vi "SHA256_hash.vi"(8 "error in (no error)":errorcluster, 11 "text in":string) -> (0 "error out":errorcluster, 3 "hash out":string)   [LabVIEW 2020]
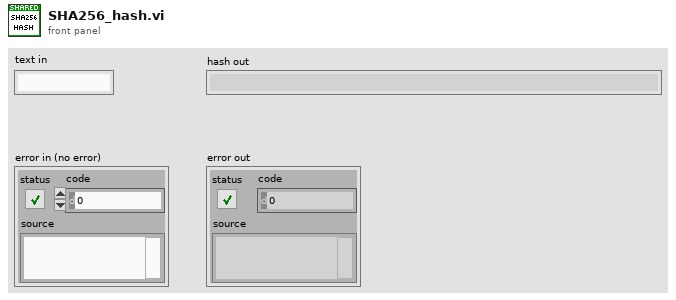
[diagram p1: front panel]
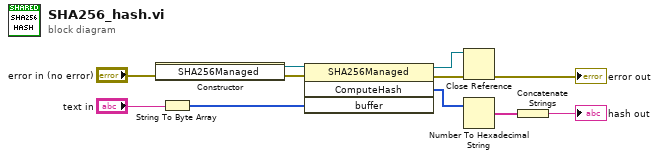
[diagram p0: block diagram]
diagram:
  n1 = constructor class="SHA256Managed"(error in="error in (no error)") -> (reference out=w9:refnum<k24>, error out=w8:errorcluster)  [unwired: 2 in, 1 out]
  n2 = String To Byte Array(string="text in") -> (unsigned byte array=w6:u8[])
  n3 = invoke class="SHA256Managed" method="ComputeHash"(reference=w9, error in=w8, "buffer"=w6) -> (reference out=w3:refnum<k24>, error out=w4:errorcluster, "ComputeHash"=w5:u8[])  [unwired: 1 in, 1 out]
  n4 = Close Reference(reference=w3, error in (no error)=w4) -> (error out=→"error out":errorcluster)
  n5 = Number To Hexadecimal String(2:w5) -> (0:w11:string[])  [unwired: 1 in]
  n6 = Concatenate Strings(w11) -> (→"hash out":string)
